vi "Telemetry Loop.vi"(6 "error in (no error)":errorcluster) -> ()   [LabVIEW 2019]
uses:
  ADIS16470/Typedef/ADIS16470 Hardware Configuration.ctl
  <vilib>/Rock Robotics/WPI/SPI/WPI_SPIMode.ctl
  <vilib>/Rock Robotics/SystemInterfaces/DIO/FPGA_DIOChannel.ctl
  <vilib>/Rock Robotics/SystemInterfaces/spilib/spi_bus.ctl
  ADIS16470/Typedef/ADIS16470 Calibration Time.ctl
  Typedef/Velocity Data.ctl
  Typedef/Odometry.ctl
  <vilib>/Rock Robotics/WPI/ThirdParty/WPILib Extensions/Geometry/Typedef/Pose2d.ctl
  <vilib>/Rock Robotics/WPI/ThirdParty/WPILib Extensions/Geometry/Typedef/Translation2d.ctl
  <vilib>/Rock Robotics/WPI/ThirdParty/WPILib Extensions/Geometry/Typedef/Rotation2d.ctl
  Drive/Pure Pursuit/Typedef/Pure Pursuit Telemetry.ctl
  Drive/Pure Pursuit/Typedef/Path Point.ctl
  <vilib>/Rock Robotics/Network Tables/NT Write Number.vi
  <vilib>/Rock Robotics/Network Tables/NT Write Numeric Array.vi
  Drive/Pure Pursuit/Visualization/Current Path.vi
  <vilib>/Rock Robotics/WPI/Counter/WPI_CounterDigitalInputToDigitalSource.vi
  Drive/Pure Pursuit/Pure Pursuit.lvlib
panel:
  in  "ADIS16470 Config":T1={"SPI Clock Rate (Hz)"=2000000.0, "IMU SPI Mode (3)"=enum."Mode 3 (Clk Idle High,Sample on Trailing)", "IMU Reset Pin"=enum."SPI Port CS2", "IMU SPI Bus"=enum."SPI On-Board, CS0", "IMU Data Ready Pin"=enum."SPI Port CS1", "Stall Config"={"Pow2BytesPerRead"=1, "StallTicks"=1000, "CsToSclkTicks"=5}}
  out "Late Iterations":i16
  out "XY Graph":cluster{dbl[], dbl[]}[](graph)=[{array[1000 elements], array[1000 elements]}, {[-2.247939211922799, 9.450601976465425, 8.114176327244312, -3.5843648611439116, -2.247939211922799], [3.8835413402382706, 1.2106900417960451, -4.638580552398066, -1.9657292539558406, 3.8835413402382706]}, {[0.0, 40.0, 60.0, 100.0], [0.0, 20.0, 80.0, 40.0]}, {array[304 elements], array[304 elements]}, {[7.524752475247524, 1.9801980198019802], [-4.118238955689372, -1.1545613507952672]}, {[-5.727080057823512, -5.705598316147173, -5.641285533198998, -5.534538218672029, -5.386014505257412, -5.196630091037495, -4.967552593902651, -4.700194352798713, -4.396203720187724, -4.057454899406876, -3.686036389581695, -3.28423810933444, -2.8545372786743237, -2.3995831461123918, -1.922180655163488, -1.4252731509367513, -0.9119242334342519, -0.38529886943823066, 0.15135612056157366, 0.6947320800959187, 1.241478915683433, 1.7882257512709472, 2.331601710805292, 2.8682567008050963, 3.3948820648011178, 3.9082309823036177, 4.405138486530354, 4.882540977479257, 5.337495110041189, 5.767195940701306, 6.16899422094856, 6.540412730773742, 6.87916155155459, 7.1831521841655785, 7.450510425269517, 7.679587922404362, 7.86897233662428, 8.017496050038897, 8.124243364565864, 8.18855614751404, 8.210037889190378, 8.18855614751404, 8.124243364565865, 8.017496050038897, 7.86897233662428, 7.679587922404362, 7.450510425269517, 7.18315218416558, 6.879161551554592, 6.540412730773744, 6.168994220948562, 5.76719594070131, 5.337495110041191, 4.882540977479256, 4.405138486530356, 3.9082309823036216, 3.3948820648011195, 2.868256700805095, 2.3316017108052938, 1.788225751270952, 1.2414789156834347, 0.6947320800959172, 0.15135612056157544, -0.3852988694382258, -0.9119242334342501, -1.4252731509367527, -1.9221806551634866, -2.3995831461123878, -2.854537278674323, -3.2842381093344417, -3.686036389581693, -4.057454899406872, -4.396203720187724, -4.700194352798713, -4.967552593902649, -5.196630091037493, -5.386014505257412, -5.534538218672031, -5.641285533198998, -5.705598316147173, -5.727080057823512], [-7.13175642584397, -7.6785032614314845, -8.22187922096583, -8.758534210965633, -9.285159574961655, -9.798508492464155, -10.295415996690892, -10.772818487639794, -11.227772620201726, -11.657473450861843, -12.059271731109098, -12.430690240934279, -12.769439061715127, -13.073429694326116, -13.340787935430054, -13.5698654325649, -13.759249846784815, -13.907773560199434, -14.0145208747264, -14.078833657674576, -14.100315399350915, -14.078833657674576, -14.0145208747264, -13.907773560199434, -13.759249846784817, -13.5698654325649, -13.340787935430054, -13.073429694326116, -12.769439061715127, -12.430690240934279, -12.0592717311091, -11.657473450861843, -11.227772620201728, -10.772818487639796, -10.295415996690892, -9.798508492464155, -9.285159574961655, -8.758534210965635, -8.22187922096583, -7.678503261431485, -7.131756425843971, -6.5850095902564565, -6.041633630722112, -5.504978640722308, -4.978353276726287, -4.465004359223786, -3.9680968549970497, -3.4906943640481467, -3.035740231486214, -2.6060394008260976, -2.2042411205788426, -1.8328226107536638, -1.4940737899728127, -1.1900831573618227, -0.922724916257887, -0.6936474191230433, -0.504263004903124, -0.355739291488506, -0.2489919769615394, -0.18467919401336363, -0.16319745233702498, -0.18467919401336363, -0.24899197696153852, -0.355739291488506, -0.5042630049031231, -0.6936474191230424, -0.9227249162578861, -1.1900831573618218, -1.4940737899728118, -1.832822610753662, -2.2042411205788417, -2.6060394008260923, -3.035740231486211, -3.4906943640481467, -3.9680968549970475, -4.465004359223782, -4.978353276726283, -5.5049786407223085, -6.041633630722109, -6.585009590256451, -7.131756425843968]}]
  out "Drivetrain Chart":T5(graph)
  out "Gyro":dbl(graph)
  out "Encoders":T6(graph)
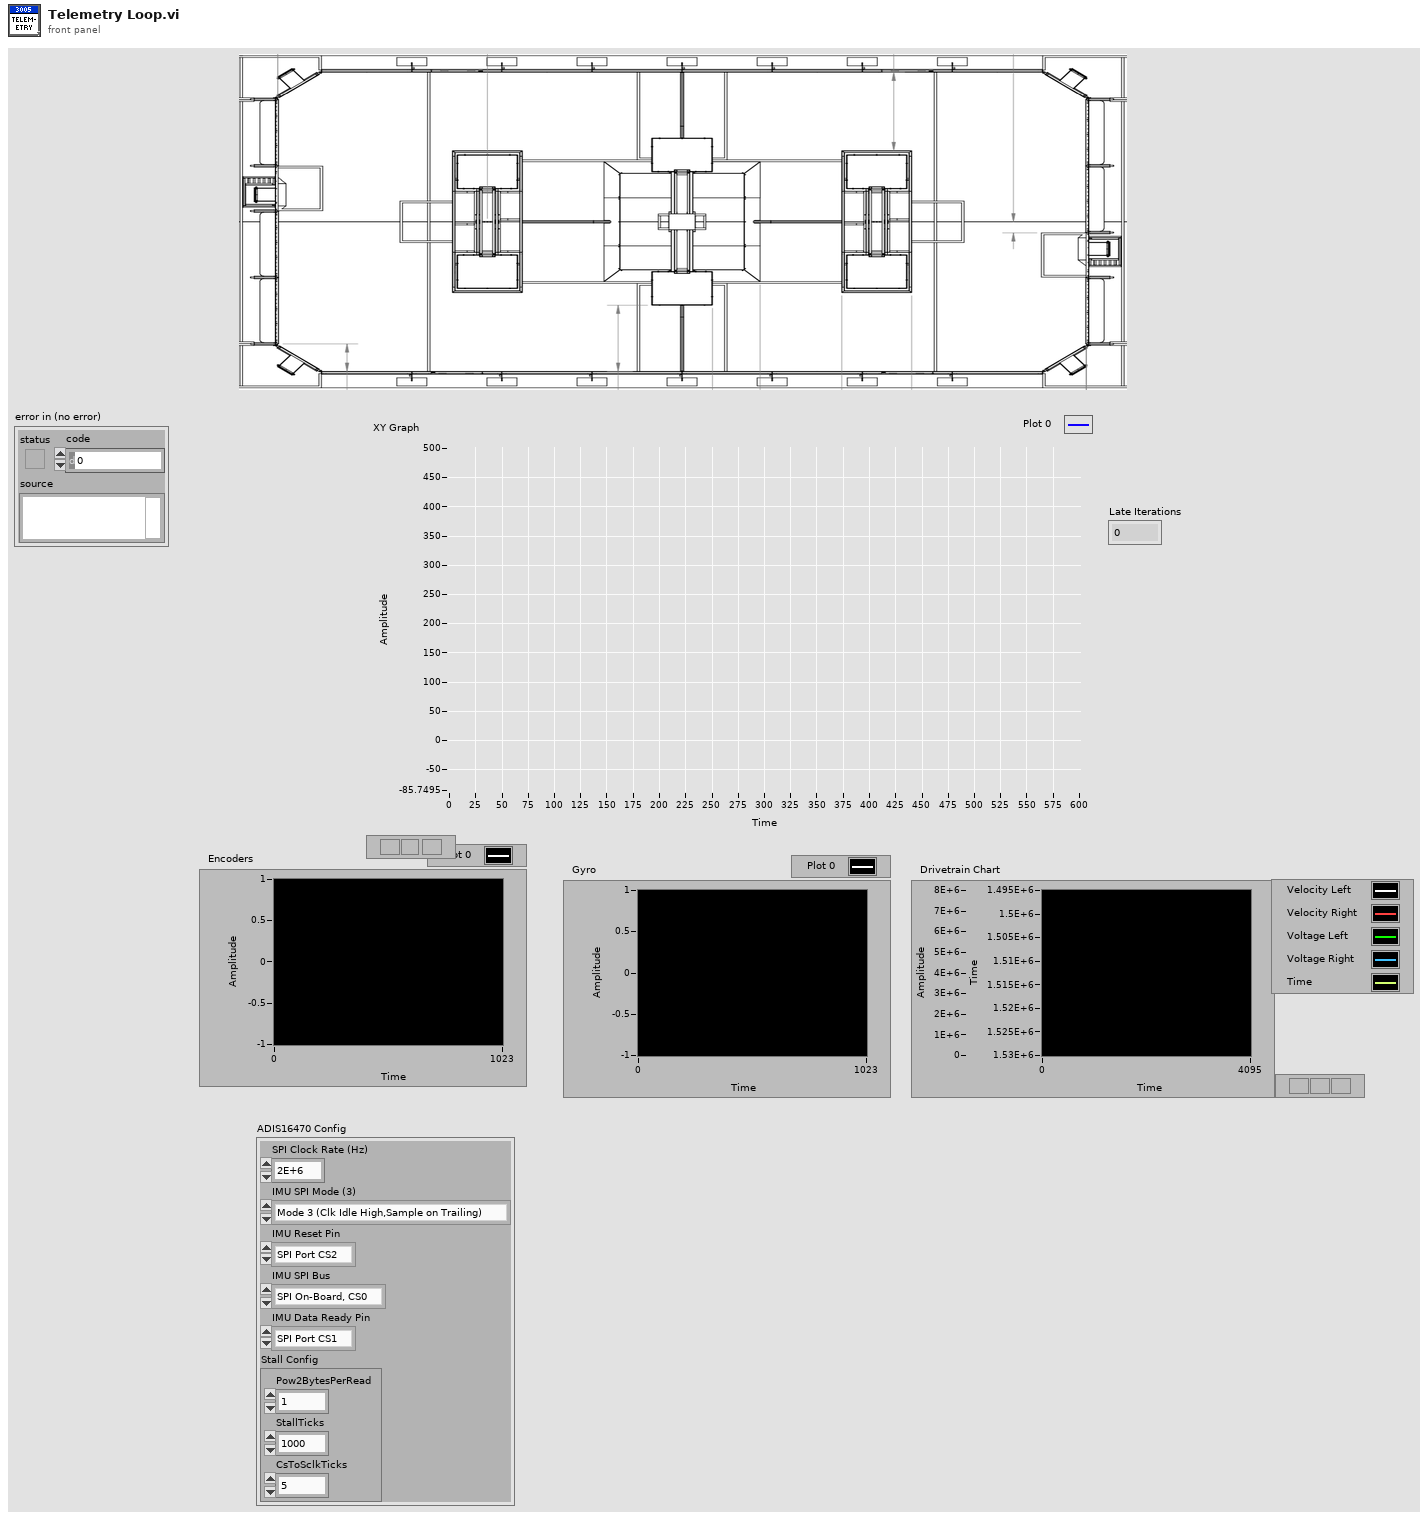
[diagram p1: front panel]
types:
  T1 = typedef "ADIS16470 Hardware Configuration.ctl" = cluster{"SPI Clock Rate (Hz)":dbl, "IMU SPI Mode (3)":T2, "IMU Reset Pin":T3, "IMU SPI Bus":T4, "IMU Data Ready Pin":T3, "Stall Config":cluster{"Pow2BytesPerRead":u8, "StallTicks":u16, "CsToSclkTicks":u8}}
  T2 = typedef "WPI_SPIMode.ctl" = enum16{"Mode 0 (Clk Idle Low,Sample on Leading)", "Mode 1 (Clk Idle Low,Sample on Trailing)", "Mode 2 (Clk Idle High,Sample on Leading)", "Mode 3 (Clk Idle High,Sample on Trailing)"}
  T3 = typedef "FPGA_DIOChannel.ctl" = enum8{"DIO 0", "DIO 1", "DIO 2", "DIO 3", "DIO 4", "DIO 5", "DIO 6", "DIO 7", "DIO 8", "DIO 9", "DIO MXP 0", "DIO MXP 1", "DIO MXP 2", "DIO MXP 3", "DIO MXP 4", "DIO MXP 5", "DIO MXP 6", "DIO MXP 7", "DIO MXP 8", "DIO MXP 9", "DIO MXP 10", "DIO MXP 11", "DIO MXP 12", "DIO MXP 13", "DIO MXP 14", "DIO MXP 15", "SPI Port CS1", "SPI Port CS2", "SPI Port CS3", "SPI Port MISO", "SPI Port MOSI", "Invalid"}
  T4 = typedef "spi_bus.ctl" = enum16{"SPI On-Board, CS0", "SPI On-Board, CS1", "SPI On-Board, CS2", "SPI On-Board, CS3", "SPI MXP", "Invalid"}
  T5 = cluster{"Left Velocity Raw":sgl, "Right Velocity Raw":sgl, "Voltage":dbl, "Voltage":dbl, "Tick Count(mSec)":u32}
  T6 = cluster{"Left Velocity Raw":sgl, "Right Velocity Raw":sgl}
  T7 = typedef "ADIS16470 Calibration Time.ctl" = enum16{"32ms", "64ms", "128ms", "256ms", "512ms", "1s", "2s", "4s", "8s", "16s", "32s", "64s"}
  T8 = typedef "WPI_DigitalInputDevRef.ctl" = cluster{"DevStatus":errorcluster, "DIO Channel":T3}
  T9 = typedef "FPGA_CounterEncoderSourceConvertionLVSourceType.ctl" = cluster{"DevStatus":errorcluster, "AnalogTriggerMode?":bool, "DigitalMode":cluster{"DIO Channel":T10}, "AnalogTriggerMode":cluster{"AnalogTriggerIndex":T11, "OutputType":T12}}
  T10 = typedef "FPGA_DIODigitalSourceChannel.ctl" = enum8{"DIO 0", "DIO 1", "DIO 2", "DIO 3", "DIO 4", "DIO 5", "DIO 6", "DIO 7", "DIO 8", "DIO 9", "DIO MXP 0", "DIO MXP 1", "DIO MXP 2", "DIO MXP 3", "DIO MXP 4", "DIO MXP 5", "DIO MXP 6", "DIO MXP 7", "DIO MXP 8", "DIO MXP 9", "DIO MXP 10", "DIO MXP 11", "DIO MXP 12", "DIO MXP 13", "DIO MXP 14", "DIO MXP 15", "SPI Port CS1", "SPI Port CS2", "SPI Port CS3", "SPI Port MISO", "SPI Port MOSI", "Disabled"}
  T11 = typedef "FPGA_AnalogTriggerIndex.ctl" = enum8{"Trig 0", "Trig 1", "Trig 2", "Trig 3", "Trig 4", "Trig 5", "Trig 6", "Trig 7", "Invalid"}
  T12 = typedef "FPGA_AnalogTriggerOutType.ctl" = enum16{"InWindow", "TriggerState", "Rising", "Falling"}
  T13 = typedef "WPI_EncoderDevRef.ctl" = cluster{"DevStatus":errorcluster, "EncoderIndex":T14, "CounterIndex":T15, "DistancePerCount":dbl, "Decoding Type":T16}
  T14 = typedef "FPGA_EncoderIdx.ctl" = enum8{"Enc 0", "Enc 1", "Enc 2", "Enc 3", "Enc 4", "Enc 5", "Enc 6", "Enc 7", "Invalid"}
  T15 = typedef "FPGA_CounterCtrSystemIndex.ctl" = enum8{"Ctr 0", "Ctr 1", "Ctr 2", "Ctr 3", "Ctr 4", "Ctr 5", "Ctr 6", "Ctr 7", "Invalid"}
  T16 = typedef "WPI_EncoderType.ctl" = enum16{"1x", "2x", "4x"}
  T17 = typedef "ADIS16470 Device Reference.ctl" = cluster{"DevStatus":errorcluster, "Hardware Config":T1, "Calibration Complete":refnum<notifier>, "Status FIFO":refnum<k33>, "Last Value Reference":refnum<data-value>, "Sychronous Process VI":T18, "Cmd FIFO":refnum<k33>, "Source":T9, "Data FIFO":refnum<k33>, "Calibration Time":T7}
  T18 = typedef "ADIS16470 Process.ctl" = refnum<vi>
  T19 = typedef "SPARKMAX6Motor.ctl" = cluster{"FrontLeftMaster":T20, "FrontLeftSlave1":T20, "FrontLeftSlave2":T20, "FrontRightMaster":T20, "FrontRightSlave1":T20, "FrontRightSlave2":T20}
  T20 = typedef "WPI_MotorControlDeviceRef.ctl" = cluster{"DeviceStatus":errorcluster, "Type":T21, "PWM":cluster{"PWM Channel":T22, "DeadBand":T23}, "CAN":cluster{"Device Number":u8, "SetOutput VI Ref":variant, "GetOutput VI Ref":variant, "Enable VI Ref":variant, "Disable VI Ref":variant, "Data":variant}, "Invert":bool, "DIO PWM":cluster{"PWM \"Enable\" Channel":T22, "DIOChannel":T3, "PWM Rate":dbl}}
  T21 = typedef "WPI_MotorControlType.ctl" = enum16{"PWM", "CAN", "DIO PWM"}
  T22 = typedef "FPGA_DIOPWMChannel.ctl" = enum8{"PWM 0", "PWM 1", "PWM 2", "PWM 3", "PWM 4", "PWM 5", "PWM 6", "PWM 7", "PWM 8", "PWM 9", "PWM MXP 0", "PWM MXP 1", "PWM MXP 2", "PWM MXP 3", "PWM MXP 4", "PWM MXP 5", "PWM MXP 6", "PWM MXP 7", "PWM MXP 8", "PWM MXP 9", "Invalid"}
  T23 = typedef "WPI_PWMDeadband.ctl" = cluster{"Name":string, "maxPositivePwm":i32, "minPositivePwm":i32, "centerPwm":i32, "maxNegativePwm":i32, "minNegativePwm":i32, "angularRange":u16}
  T24 = typedef "Pure Pursuit.lvlib/Pure Pursuit Telemetry.ctl" = cluster{"Target Point":T25, "Close Point":T25, "Curvature":dbl, "index out":i32}
  T25 = typedef "Pure Pursuit.lvlib/Path Point.ctl" = cluster{"x":dbl, "y":dbl, "heading":dbl, "curvature":dbl, "total distance":dbl, "velocity expected":dbl}
  T26 = typedef "Odometry.ctl" = cluster{"Left Encoder":dbl, "Right Encoder":dbl, "Late Iterations":i16, "Pose2d":T27}
  T27 = typedef "Pose2d.ctl" = cluster{"Translation2d":T28, "Rotation2d":T29}
  T28 = typedef "Translation2d.ctl" = cluster{"x":dbl, "y":dbl}
  T29 = typedef "Rotation2d.ctl" = cluster{"Theta":dbl}
  T30 = typedef "Velocity Data.ctl" = cluster{"Right Velocity Raw":sgl, "Left Velocity Raw":sgl}
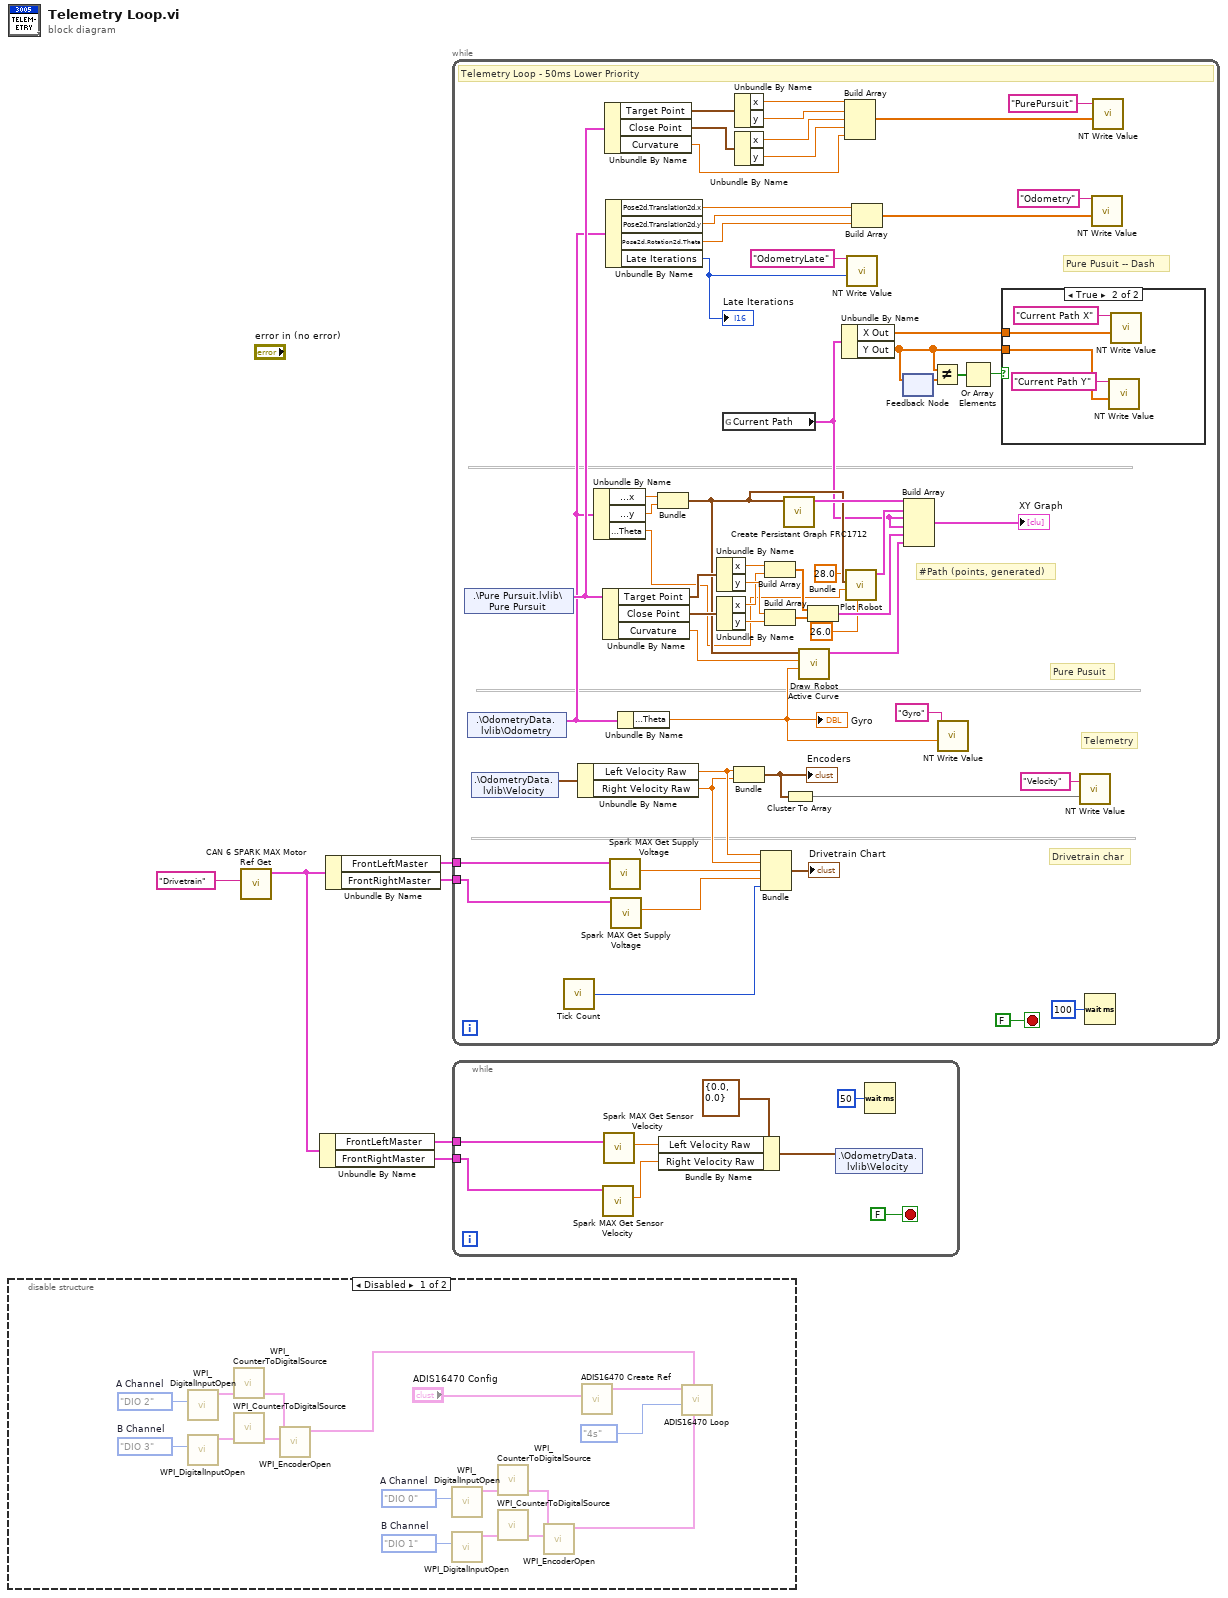
[diagram p0: block diagram]
diagram:
  n1 = disable-structure shown="Disabled" {
    frame Disabled {
      w8 = FPGA_DIOChannel."DIO 3"  # B Channel
      w9 = FPGA_DIOChannel."DIO 2"  # A Channel
      w20 = FPGA_DIOChannel."DIO 1"  # B Channel
      w19 = FPGA_DIOChannel."DIO 0"  # A Channel
      n2 = call <vilib>:"WPI_DigitalInputOpen.vi"("DIO Channel"=w9) -> ("DigitalInputDevRef"=w12:T8)  [unwired: 1 in, 9 out]
      n3 = call <vilib>:"WPI_DigitalInputOpen.vi"("DIO Channel"=w8) -> ("DigitalInputDevRef"=w11:T8)  [unwired: 1 in, 9 out]
      n4 = call-poly <vilib>:"WPI_CounterToDigitalSource.vi"("DigitalInputDevRef"=w12) -> ("Digital Source"=w13:T9)  [unwired: 6 out]
      n5 = call-poly <vilib>:"WPI_CounterToDigitalSource.vi"("DigitalInputDevRef"=w11) -> ("Digital Source"=w10:T9)  [unwired: 6 out]
      n6 = call <vilib>:"WPI_EncoderOpen.vi"("BSource"=w10, "ASource"=w13) -> ("EncoderDevRef"=w7:T13)  [unwired: 6 in, 3 out]
      n7 = call <vilib>:"WPI_DigitalInputOpen.vi"("DIO Channel"=w19) -> ("DigitalInputDevRef"=w16:T8)  [unwired: 1 in, 9 out]
      n8 = call <vilib>:"WPI_DigitalInputOpen.vi"("DIO Channel"=w20) -> ("DigitalInputDevRef"=w17:T8)  [unwired: 1 in, 9 out]
      n9 = call-poly <vilib>:"WPI_CounterToDigitalSource.vi"("DigitalInputDevRef"=w16) -> ("Digital Source"=w15:T9)  [unwired: 6 out]
      n10 = call-poly <vilib>:"WPI_CounterToDigitalSource.vi"("DigitalInputDevRef"=w17) -> ("Digital Source"=w18:T9)  [unwired: 6 out]
      n11 = call <vilib>:"WPI_EncoderOpen.vi"("BSource"=w18, "ASource"=w15) -> ("EncoderDevRef"=w14:T13)  [unwired: 6 in, 3 out]
      n12 = call "ADIS16470 Create Ref.vi"("Hardware Config"="ADIS16470 Config") -> ("ADIS16470DevRef"=w23:T17)  [unwired: 9 in, 1 out]
      n13 = call "ADIS16470 Loop.vi"("Encoder R"=w14, "Encoder L"=w7, "Calibration Time"=ADIS16470_Calibration_Time."4s", "ADIS16470DevRef"=w23) -> ()  [unwired: 8 in]
    }
    frame Enabled {
    }
  }
  n14 = call "CAN 6 SPARK MAX Motor Ref Get.vi"("refnum name"="Drivetrain") -> ("TalonSRX6MotorRef out"=w3:T19)  [unwired: 9 in, 1 out]
  n15 = Unbundle By Name(w3) -> ("FrontLeftMaster"=w2:T20, "FrontRightMaster"=w1:T20)
  n16 = Unbundle By Name(w3) -> ("FrontLeftMaster"=w5:T20, "FrontRightMaster"=w4:T20)
  n17 = while {
    tunnel: w5 -> [w30]
    tunnel: w4 -> [w27]
    stop <- FALSE stop-if-true
    # "Pure Pusuit -- Dash"
    # "Telemetry"
    # "Drivetrain char"
    # "Pure Pusuit"
    # "#Path (points, generated)"
    # "Telemetry Loop - 50ms Lower Priority"
    n18 = shared-variable ".\\Pure Pursuit.lvlib\\Pure Pursuit"() -> (w52:T24)  [unwired: 1 in, 1 out]
    n19 = shared-variable ".\\OdometryData.lvlib\\Odometry"() -> (w43:T26)  [unwired: 1 in, 1 out]
    n20 = shared-variable ".\\OdometryData.lvlib\\Velocity"() -> (w26:T30)  [unwired: 1 in, 1 out]
    n21 = call "Tick Count"() -> ("Tick Count(mSec)"=w58:u32)
    n22 = Unbundle By Name(w26) -> ("Left Velocity Raw"=w25:sgl, "Right Velocity Raw"=w24:sgl)
    n23 = Unbundle By Name(w43) -> ("Pose2d.Translation2d.x"=w78:dbl, "Pose2d.Translation2d.y"=w77:dbl, "Pose2d.Rotation2d.Theta"=w60:dbl)
    n24 = Unbundle By Name(w52) -> ("Target Point"=w67:T25, "Close Point"=w66:T25, "Curvature"=w65:dbl)
    n25 = Unbundle By Name(w52) -> ("Target Point"=w51:T25, "Close Point"=w50:T25, "Curvature"=w45:dbl)
    n26 = Unbundle By Name(w43) -> ("Pose2d.Translation2d.x"=w42:dbl, "Pose2d.Translation2d.y"=w41:dbl, "Pose2d.Rotation2d.Theta"=w40:dbl, "Late Iterations"=w31:i16)
    "Late Iterations" <- w31
    n27 = call <vilib>:"Spark MAX Get Supply Voltage.vi"("MotorControlDevRef in"=w30) -> ("Voltage"=w29:dbl)  [unwired: 7 in, 3 out]
    n28 = call <vilib>:"Spark MAX Get Supply Voltage.vi"("MotorControlDevRef in"=w27) -> ("Voltage"=w28:dbl)  [unwired: 7 in, 3 out]
    n29 = Unbundle By Name(w43) -> ("Pose2d.Rotation2d.Theta"=w63:dbl)
    "Gyro" <- w63
    n30 = Bundle("x"=w78, "y"=w77) -> (w62:cluster{"x":dbl, "y":dbl})  [unwired: 1 in]
    n31 = Unbundle By Name(w67) -> ("x"=w74:dbl, "y"=w73:dbl)
    n32 = Unbundle By Name(w66) -> ("x"=w70:dbl, "y"=w69:dbl)
    n33 = global read "Current Path.vi" "Current Path"() -> (w38:cluster{"X Out":dbl[], "Y Out":dbl[]})
    n34 = Bundle("Left Velocity Raw"=w25, "Right Velocity Raw"=w24) -> (w56:T6)  [unwired: 1 in]
    "Encoders" <- w56
    n35 = Unbundle By Name(w51) -> ("x"=w49:dbl, "y"=w48:dbl)
    n36 = Unbundle By Name(w50) -> ("x"=w47:dbl, "y"=w46:dbl)
    n37 = Bundle("Left Velocity Raw"=w25, "Right Velocity Raw"=w24, "Voltage"=w29, "Voltage"=w28, "Tick Count(mSec)"=w58) -> (→"Drivetrain Chart":T5)  [unwired: 1 in]
    n38 = Build Array(w74, w70) -> (w71:dbl[])
    n39 = Build Array(w73, w69) -> (w72:dbl[])
    n40 = call "Create Persistant Graph FRC1712.vi"("XY"=w62) -> ("Graph Plot"=w81:cluster{dbl[], dbl[]})  [unwired: 10 in]
    n41 = Cluster To Array(cluster=w56) -> (array=w55:sgl[])
    n42 = call "Draw Robot Active Curve.vi"("theta"=w63, "Curvature"=w65, "Cluster"=w62) -> ("circle"=w64:cluster{dbl[], dbl[]})  [unwired: 8 in]
    n43 = Bundle(w71, w72) -> (w68:cluster{dbl[], dbl[]})  [unwired: 1 in]
    n44 = Unbundle By Name(w38) -> ("X Out"=w37:dbl[], "Y Out"=w35:dbl[])
    n45 = Build Array(w49, w48, w47, w46, w45) -> (w44:dbl[])
    n46 = call "Plot Robot.vi"("Length"=26.0, "Angle"=w60, "Location"=w62, "Width"=28.0) -> ("Cluster"=w75:cluster{"X Out":dbl[], "Y Out":dbl[]})  [unwired: 7 in]
    n47 = call-poly <vilib>:"NT Write Value.vi"("Numeric"=w31, "Name"="OdometryLate") -> ()  [unwired: 9 in, 1 out]
    n48 = Build Array(w42, w41, w40) -> (w39:dbl[])
    n49 = feedback-in #1(w35) -> ()
    n50 = feedback #1() -> (w36:dbl[])  [unwired: 1 in]
    n51 = Build Array(w81, w75, w38, w38, w68, w64) -> (→"XY Graph":cluster{"X Out":dbl[], "Y Out":dbl[]}[])
    n52 = Not Equal?(x=w35, y=w36) -> (x != y?=w34:bool[])
    n53 = call-poly <vilib>:"NT Write Value.vi"("Numeric"=w63, "Name"="Gyro") -> ()  [unwired: 9 in, 1 out]
    n54 = Or Array Elements(Boolean array=w34) -> (logical OR=w33:bool)
    n55 = case shown="True" w33 {
      tunnel: w35 -> [_ w85]
      tunnel: w37 -> [_ w84]
      frame False {
      }
      frame True {
        n56 = call-poly <vilib>:"NT Write Value.vi"("Numeric Array"=w85, "Name"="Current Path Y") -> ()  [unwired: 9 in, 1 out]
        n57 = call-poly <vilib>:"NT Write Value.vi"("Numeric Array"=w84, "Name"="Current Path X") -> ()  [unwired: 9 in, 1 out]
      }
    }
    n58 = call-poly <vilib>:"NT Write Value.vi"("Numeric Array"=w55, "Name"="Velocity") -> ()  [unwired: 9 in, 1 out]
    n59 = Wait (ms)(milliseconds to wait=u32 100) -> ()  [unwired: 1 out]
    n60 = call-poly <vilib>:"NT Write Value.vi"("Numeric Array"=w39, "Name"="Odometry") -> ()  [unwired: 9 in, 1 out]
    n61 = call-poly <vilib>:"NT Write Value.vi"("Numeric Array"=w44, "Name"="PurePursuit") -> ()  [unwired: 9 in, 1 out]
  }
  n62 = while {
    tunnel: w2 -> [w93]
    tunnel: w1 -> [w92]
    stop <- FALSE stop-if-true
    n63 = call <vilib>:"Spark MAX Get Sensor Velocity.vi"("MotorControlDevRef in"=w92) -> ("Sensor Velocity"=w91:dbl)  [unwired: 7 in, 3 out]
    n64 = call <vilib>:"Spark MAX Get Sensor Velocity.vi"("MotorControlDevRef in"=w93) -> ("Sensor Velocity"=w90:dbl)  [unwired: 7 in, 3 out]
    n65 = Bundle By Name(cluster=T30 {"Right Velocity Raw"=0.0, "Left Velocity Raw"=0.0} ("Velocity"), "Left Velocity Raw"=w90, "Right Velocity Raw"=w91) -> (w89:T30)
    n66 = shared-variable ".\\OdometryData.lvlib\\Velocity"(w89) -> ()  [unwired: 1 in, 1 out]
    n67 = Wait (ms)(milliseconds to wait=u32 50) -> ()  [unwired: 1 out]
  }
